vi "Error Type to Error Cluster.vi"(0 "VIAn Error":T1, 5 "details":string) -> (15 "error out":errorcluster)   [LabVIEW 2020]
uses:
  <vilib>/addons/analyzer/Typedefs/VIAn Error Description.ctl
  <vilib>/ErrorRing/Error Ring.xnode
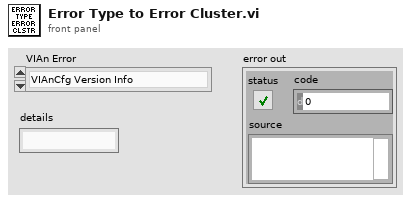
[diagram p1: front panel]
types:
  T1 = typedef "VIAn Error Description.ctl" = enum16{"VIAnCfg Version Info", "VIAnalyzerConfiguration"}
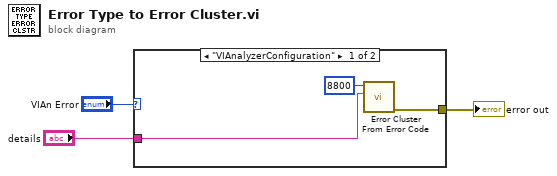
[diagram p0: block diagram]
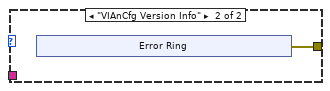
[diagram p2: hidden frame]
diagram:
  n1 = case shown="\"VIAnalyzerConfiguration\"" "VIAn Error" {
    tunnel: [w6 w7] -> w3
    tunnel: "details" -> [w4 _]
    frame "VIAnalyzerConfiguration" {
      n2 = call <vilib>:"Error Cluster From Error Code.vi"("error message (\"\")"=w4, "error code (0)"=8800) -> ("error out"=w6:errorcluster)  [unwired: 7 in]
    }
    frame "VIAnCfg Version Info" {
      n3 = xnode "Error Ring"() -> ("error out"=w7:errorcluster)
    }
  }
  "error out" <- w3
